vi "Read Scanner driver.vi"(8 "error in (no error)":errorcluster, 11 "Channel Scanner in":refnum<class "Channel Scanner.lvclass">) -> (0 "error out":errorcluster, 2 "Channel Scanner Driver.lvclass":refnum<class "Channel Scanner Driver.lvclass">, 3 "Channel Scanner out":refnum<class "Channel Scanner.lvclass">)   [LabVIEW 2016, in "Channel Scanner.lvclass"]
uses:
  Channel Scanner.lvclass
  D:/github/Measure_core/Instrument Recorders/Instrument Recorder/Instrument Recorder.lvclass
  NHMFL_Core/Libraries/Instruments/Instrument Driver/Channel Scanner Driver/Channel Scanner Driver.lvclass
  Measure_core/Instrument Recorders/Instrument Recorder/Instrument Recorder.lvclass/Instrument Recorder.ctl
  Measure_core/Instrument Recorders/Instrument Recorder/Read Instrument driver.vi
  NHMFL_Core/Libraries/Instruments/Instrument Driver/Instrument Driver.lvclass
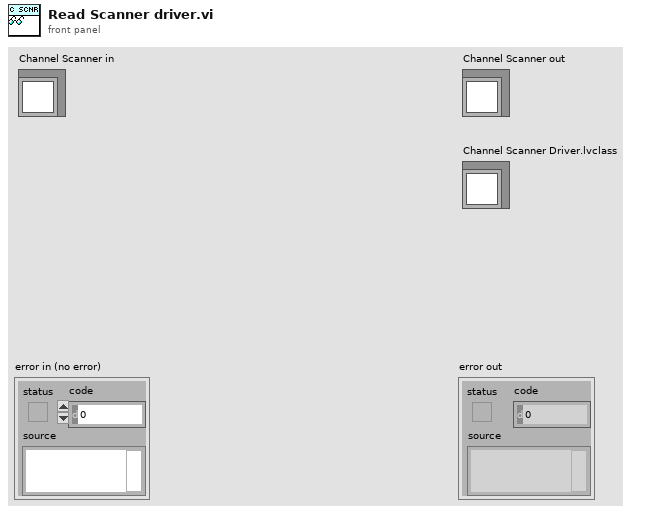
[diagram p1: front panel]
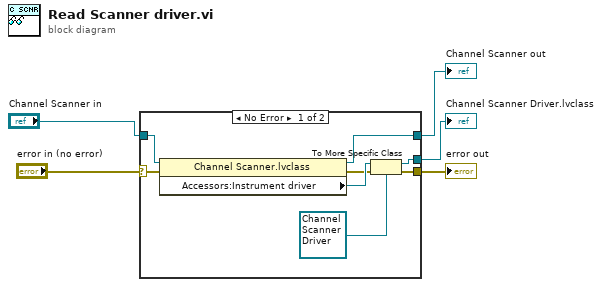
[diagram p0: block diagram]
diagram:
  n1 = case shown="No Error" "error in (no error)" {
    selector: "error in (no error)" -> [w9 w14]
    tunnel: [w8 w14] -> w4
    tunnel: [w12 w15] -> w2
    tunnel: "Channel Scanner in" -> [w13 w15]
    tunnel: [w6 _] -> w1
    frame No Error {
      n2 = property class="Channel Scanner.lvclass"(reference=w13, error in=w9) -> (reference out=w12:refnum<class "Channel Scanner.lvclass">, error out=w10:errorcluster, "Accessors:Instrument driver"=w11:refnum<class "Instrument Driver.lvclass">)
      n3 = To More Specific Class(target class=refnum<class "Channel Scanner Driver.lvclass"> refnum ("Channel Scanner Driver.lvclass"), reference=w11, error in=w10) -> (specific class reference=w6:refnum<class "Channel Scanner Driver.lvclass">, error out=w8:errorcluster)
    }
    frame Error {
    }
  }
  "error out" <- w4
  "Channel Scanner out" <- w2
  "Channel Scanner Driver.lvclass" <- w1
